vi "ProcessingLoop.vi"(8 "error in (no error)":errorcluster, 11 "navX - Interface in":refnum<class "navX - SERIAL.lvclass">) -> (0 "error out":errorcluster, 3 "navX - Interface out":refnum<class "navX - SERIAL.lvclass">)   [LabVIEW 2015, in "navX Library v3.lvlib" / "navX - SERIAL.lvclass"]
uses:
  navX - SERIAL.lvclass
  navX Error Status/navX Error Status.lvclass
  navX - Interface/navX - Interface.lvclass/navX - Interface.ctl
  navX - SERIAL.lvclass/navX - SERIAL.ctl
  navX - Interface/navX - Interface.lvclass
panel:
  out "navX - Interface internal":refnum<class "navX - SERIAL.lvclass">
  in  "Halt?":bool
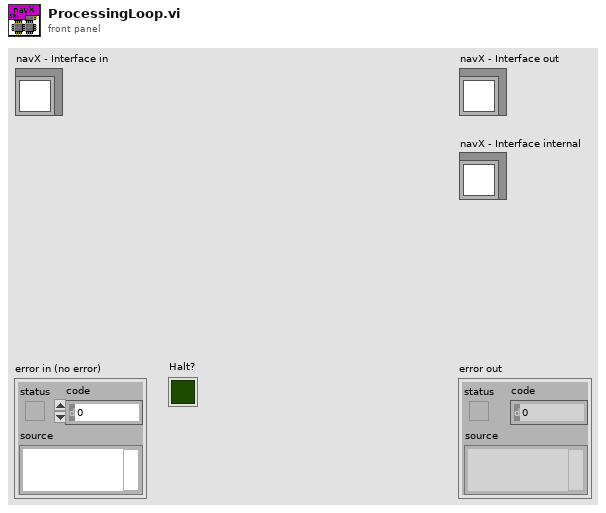
[diagram p1: front panel]
types:
  T1 = typedef "WPI_SerialPortRef.ctl" = cluster{"DevStatus":errorcluster, "Serial Port Name":refnum<visa-resource-name>}
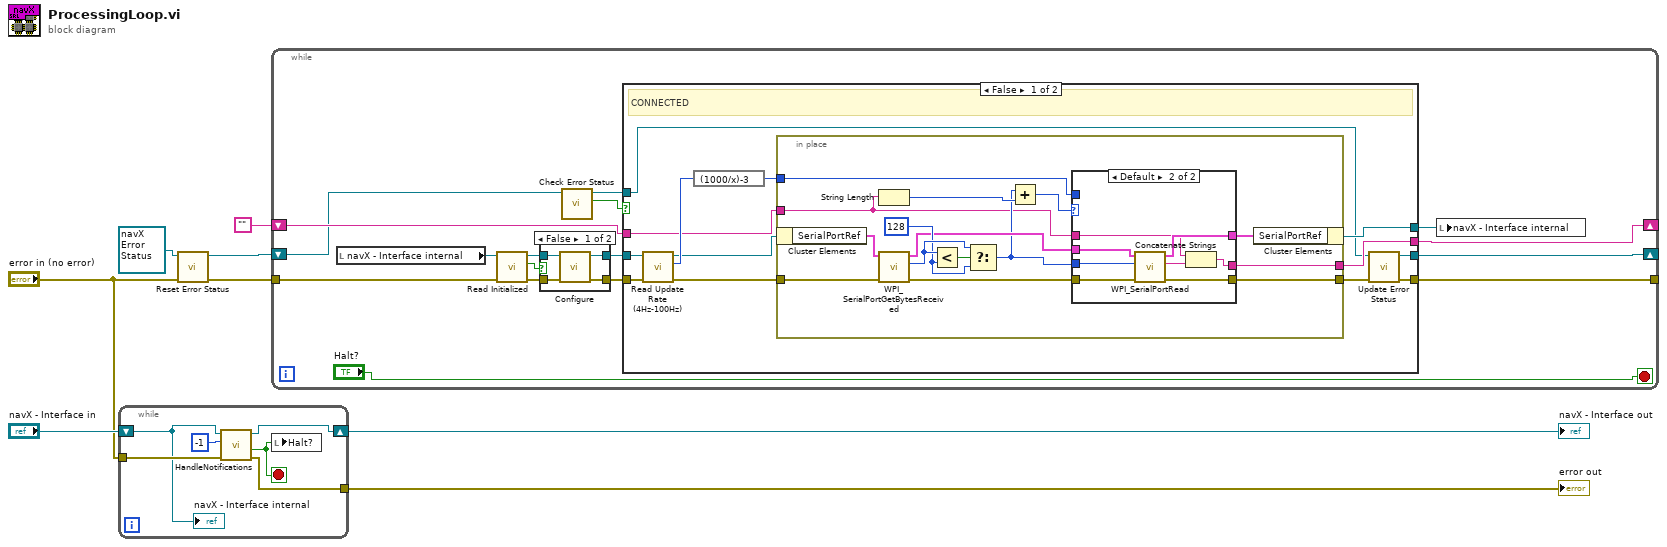
[diagram p0: block diagram]
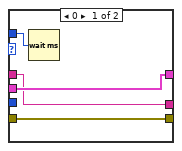
[diagram p3: hidden frame]
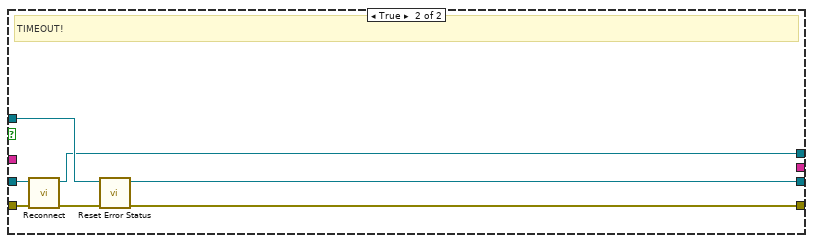
[diagram p4: hidden frame]
diagram:
  n1 = while {
    tunnel: "error in (no error)" -> [w14]
    shift-right: [w11] -> w3
    shift-left: "navX - Interface in" -> [w9]
    tunnel: [w10] -> w2
    stop <- w12 stop-if-true
    n2 = call "HandleNotifications.vi"("error in (no error)"=w14, "timeout in ms (0)"=-1, "navX - Interface in"=w9) -> ("error out"=w10:errorcluster, "Halt?"=w12:bool, "navX - Interface out"=w11:refnum<class "navX - SERIAL.lvclass">)  [unwired: 6 in]
    n3 = local write "Halt?"(w12) -> ()
    "navX - Interface internal" <- w9
  }
  "error out" <- w2
  "navX - Interface out" <- w3
  n4 = call "Reset Error Status.vi"("error in (no error)"="error in (no error)", "navX Error Status in"=refnum<class "navX Error Status.lvclass"> refnum ("navX Library v3.lvlib:navX Error Status.lvclass")) -> ("error out"=w1:errorcluster, "navX Error Status out"=w6:refnum<class "navX Error Status.lvclass">)  [unwired: 8 in]
  n5 = while {
    tunnel: w1 -> [w21]
    tunnel: [w29] -> _
    shift-right: [w27] -> _
    shift-left: "" -> [w28]
    shift-right: [w23] -> _
    shift-left: w6 -> [w26]
    stop <- "Halt?" stop-if-true
    n6 = local read "navX - Interface internal"() -> (w17:refnum<class "navX - SERIAL.lvclass">)
    n7 = call "Read Initialized.vi"("error in (no error)"=w21, "navX - Interface in"=w17) -> ("error out"=w18:errorcluster, "Initialized?"=w20:bool, "navX - Interface out"=w19:refnum<class "navX - SERIAL.lvclass">)  [unwired: 7 in]
    n8 = case shown="False" w20 {
      tunnel: [w34 w35] -> w15
      tunnel: [w33 w36] -> w16
      tunnel: w19 -> [w32 w36]
      tunnel: w18 -> [w31 w35]
      frame False {
        n9 = call-dynamic "Configure.vi"("error in (no error)"=w31, "navX - SERIAL in"=w32) -> ("error out"=w34:errorcluster, "navX - SERIAL out"=w33:refnum<class "navX - SERIAL.lvclass">)  [unwired: 8 in]
      }
      frame True {
      }
    }
    n10 = call "Check Error Status.vi"("navX Error Status in"=w26) -> ("Timeout!"=w25:bool, "navX Error Status out"=w24:refnum<class "navX Error Status.lvclass">)  [unwired: 8 in, 1 out]
    n11 = case shown="False" w25 {
      tunnel: [w49 w78] -> w22
      tunnel: [w39 w80] -> w29
      tunnel: w16 -> [w47 w79]
      tunnel: w15 -> [w45 w81]
      tunnel: w28 -> [w42 _]
      tunnel: [w41 _] -> w27
      tunnel: w24 -> [w37 w83]
      tunnel: [w38 w77] -> w23
      frame False {
        # "CONNECTED"
        n12 = call "Read Update Rate (4Hz-100Hz).vi"("error in (no error)"=w45, "navX - Interface in"=w47) -> ("error out"=w44:errorcluster, "Update Rate (4Hz-100Hz)"=w48:u8, "navX - Interface out"=w46:refnum<class "navX - SERIAL.lvclass">)  [unwired: 7 in]
        n13 = expression code="(1000/x)-3"(w48) -> (w43:u8)
        n14 = in-place {
          in-place-border: [w55] -> w40
          in-place-border: w44 -> [w56]
          in-place-border: w43 -> [w60]
          in-place-border: w42 -> [w51]
          in-place-border: [w50] -> w41
          w61 = u32 128 ("Bytes at Port")
          n15 = in-place-cluster #1(w46) -> ("SerialPortRef"=w64:T1)
          n16 = String Length(string=w51) -> (length=w54:i32)
          n17 = call <vilib>:"WPI_SerialPortGetBytesReceived.vi"("error in (no error)"=w56, "SerialPortRef"=w64) -> ("error out"=w58:errorcluster, "Bytes at Port"=w62:u32, "SerialPortRef"=w59:T1)  [unwired: 7 in]
          n18 = Less?(x=w62, y=w61) -> (x < y?=w63:bool)
          n19 = Select(t=w62, s=w63, f=w61) -> (s? t:f=w53:u32)
          n20 = Add(x=w53, y=w54) -> (x+y=w52:u32)
          n21 = case shown="Default" w52 {
            tunnel: w60 -> [w68 _]
            tunnel: w59 -> [w67 w76]
            tunnel: w58 -> [w66 w75]
            tunnel: [w66 w74] -> w55
            tunnel: [w67 w73] -> w57
            tunnel: w53 -> [_ w72]
            tunnel: w51 -> [w65 w71]
            tunnel: [w65 w69] -> w50
            frame 0 {
              n22 = Wait (ms)(milliseconds to wait=w68) -> ()  [unwired: 1 out]
            }
            frame Default {
              n23 = call <vilib>:"WPI_SerialPortRead.vi"("error in (no error)"=w75, "Num Bytes to Read"=w72, "SerialPortRef"=w76) -> ("error out"=w74:errorcluster, "Buffer"=w70:string, "SerialPortRef"=w73:T1)  [unwired: 6 in]
              n24 = Concatenate Strings(w71, w70) -> (w69:string)
            }
          }
          n25 = in-place-cluster #1("SerialPortRef"=w57) -> (w49:refnum<class "navX - SERIAL.lvclass">)
        }
        n26 = call "Update Error Status.vi"("error in (no error)"=w40, "navX Status in"=w37) -> ("error out"=w39:errorcluster, "navX Status out"=w38:refnum<class "navX Error Status.lvclass">)  [unwired: 7 in, 1 out]
      }
      frame True {
        # "TIMEOUT!"
        n27 = call-dynamic "Reconnect.vi"("error in (no error)"=w81, "navX - SERIAL in"=w79) -> ("error out"=w82:errorcluster, "navX - SERIAL out"=w78:refnum<class "navX - SERIAL.lvclass">)  [unwired: 8 in]
        n28 = call "Reset Error Status.vi"("error in (no error)"=w82, "navX Error Status in"=w83) -> ("error out"=w80:errorcluster, "navX Error Status out"=w77:refnum<class "navX Error Status.lvclass">)  [unwired: 8 in]
      }
    }
    n29 = local write "navX - Interface internal"(w22) -> ()
  }
